vi "Initialize.vi"(5 "error in (no error)":errorcluster) -> (14 "video out":refnum<class "MSC Video.lvclass">, 19 "error out":errorcluster)   [LabVIEW 2014, in "MSC Video.lvclass"]
doc: "Initializes a video."
uses:
  MSC Video.lvclass
  controls/Video.ctl
  MSC Video.lvclass/MSC Video.ctl
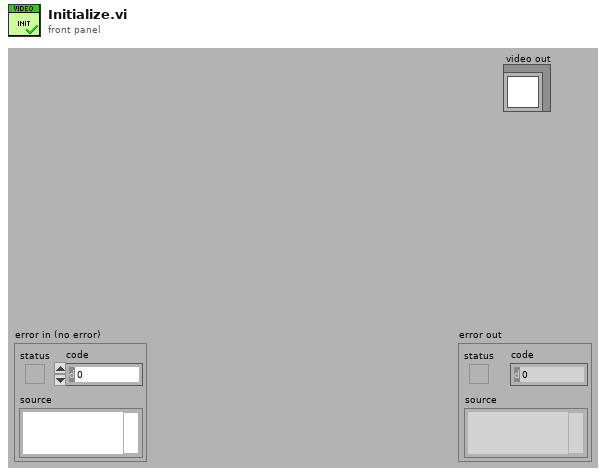
[diagram p1: front panel]
types:
  T1 = typedef "MSC Video.lvclass/Video.ctl" = cluster{"Pointer":u64, "CamID":i32, "File Path":path, "Network Address":string, "opened":bool}
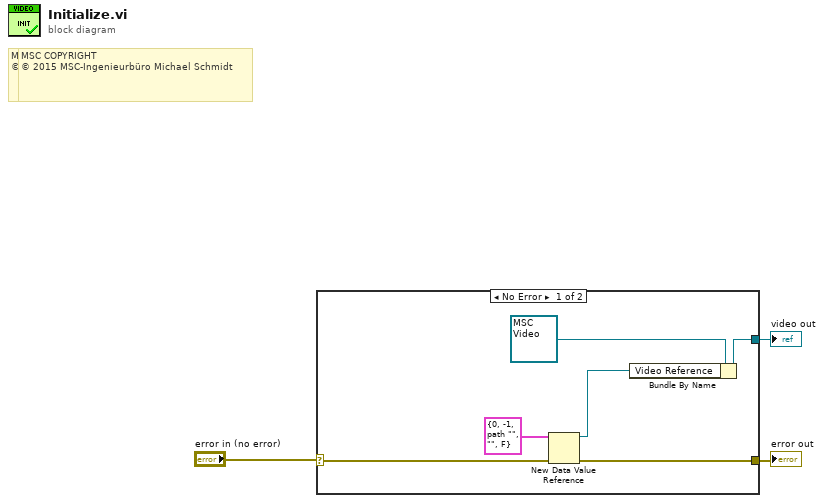
[diagram p0: block diagram]
diagram:
  # "MSC COPYRIGHT\n© 2016 MSC-Ingenieurbüro Michael Schmidt"
  # "MSC COPYRIGHT\n© 2016 MSC-Ingenieurbüro Michael Schmidt"
  # "MSC COPYRIGHT\n© 2015 MSC-Ingenieurbüro Michael Schmidt"
  n1 = case shown="No Error" "error in (no error)" {
    selector: "error in (no error)" -> [w6 w10]
    tunnel: [w9 _] -> w3
    tunnel: [w5 w10] -> w1
    frame No Error {
      n2 = New Data Value Reference(data value=T1 {"Pointer"=0, "CamID"=-1, "File Path"=path "", "Network Address"="", "opened"=FALSE}, error in=w6) -> (data value reference=w7:refnum<data-value>, error out=w5:errorcluster)
      n3 = Bundle By Name(cluster=refnum<class "MSC Video.lvclass"> refnum ("video in"), "Video Reference"=w7) -> (w9:refnum<class "MSC Video.lvclass">)
    }
    frame Error {
    }
  }
  "video out" <- w3
  "error out" <- w1
